vi "PlantModel.vi"(7 "error in (no error)":errorcluster, 8 "ROSCO Params in":T1, 9 "?":T2={"iSTATUS"=0, "TIME"=1, "DT"=2, "BL_PITCH_1"=3, "VS_MECHGENPWR"=13, "GEN_SPEED"=19, "ROT_SPEED"=20, "GENTQMEAS"=22, "Y_M"=23, "HORWINDV"=26, "ROOTMOOP1"=29, "ROOTMOOP2"=30, "BL_PITCH_2"=32, "BL_PITCH_3"=33, "ROOTMOOP3"=31, "INFILE_SIZE"=49, "FA_ACC"=52, "NUM_BLADES"=60, " OUT BL_PITCH"=44, "OUT_ TORQUE"=46, "OUTFILE_SIZE "=49, "AVCMSG_SIZE"=49, "AERODYN TQ"=89, "VS_GENPWR"=13}) -> (0 "error out":errorcluster, 1 "ROSCO Params out":T1, 3 "wdot/w":sgl)   [LabVIEW 2018]
uses:
  Clusters/RoscoParams.ctl
  Clusters/SwapIndexes.ctl
  Clusters/SimulationConstants.ctl
panel:
  out "element 4":sgl
  out "element 3":sgl
  out "element 2":sgl
  out "element":sgl
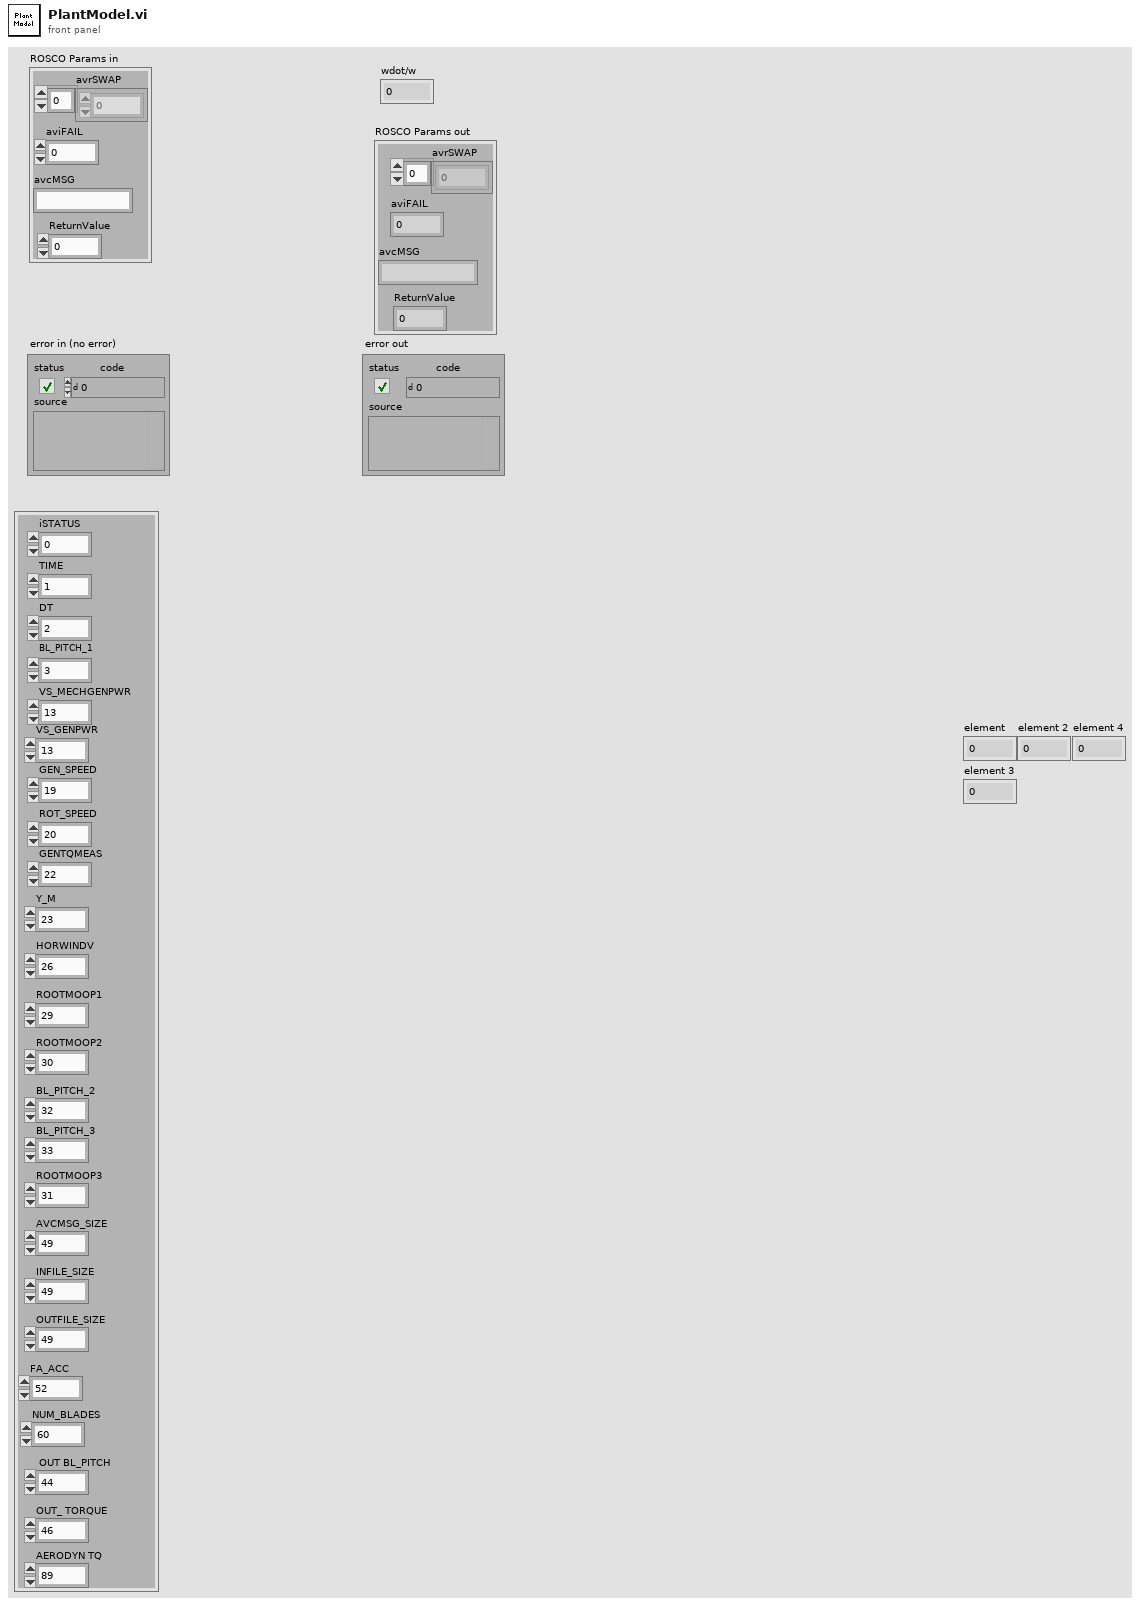
[diagram p1: front panel]
types:
  T1 = typedef "RoscoParams.ctl" = cluster{"avrSWAP":sgl[], "aviFAIL":i32, "avcMSG":string, "ReturnValue":i32}
  T2 = typedef "SwapIndexes.ctl" = cluster{"iSTATUS":i32, "TIME":i32, "DT":i32, "BL_PITCH_1":i32, "VS_MECHGENPWR":i32, "GEN_SPEED":i32, "ROT_SPEED":i32, "GENTQMEAS":i32, "Y_M":i32, "HORWINDV":i32, "ROOTMOOP1":i32, "ROOTMOOP2":i32, "BL_PITCH_2":i32, "BL_PITCH_3":i32, "ROOTMOOP3":i32, "INFILE_SIZE":i32, "FA_ACC":i32, "NUM_BLADES":i32, " OUT BL_PITCH":i32, "OUT_ TORQUE":i32, "OUTFILE_SIZE ":i32, "AVCMSG_SIZE":i32, "AERODYN TQ":i32, "VS_GENPWR":i32}
  T3 = typedef "SimulationConstants.ctl" = cluster{"Ngear":sgl, "RotorInertia":sgl, "GeneratorEff":sgl, "RotorRadius":sgl, "Rho":sgl}
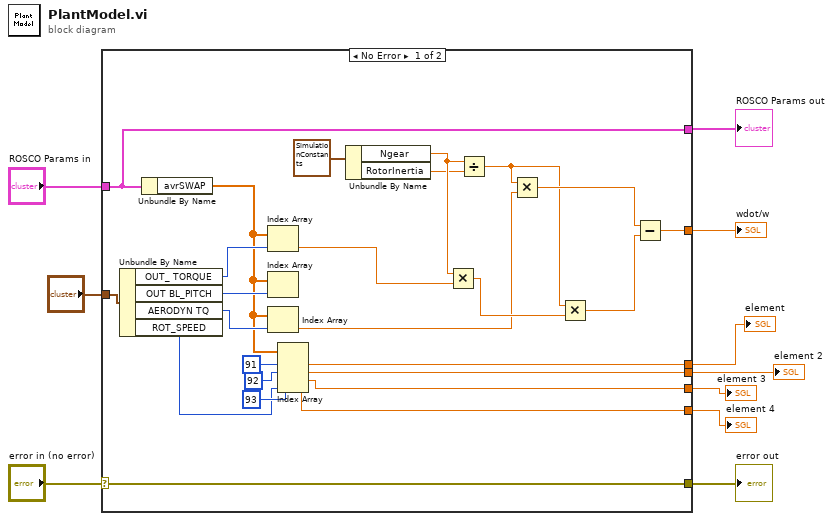
[diagram p0: block diagram]
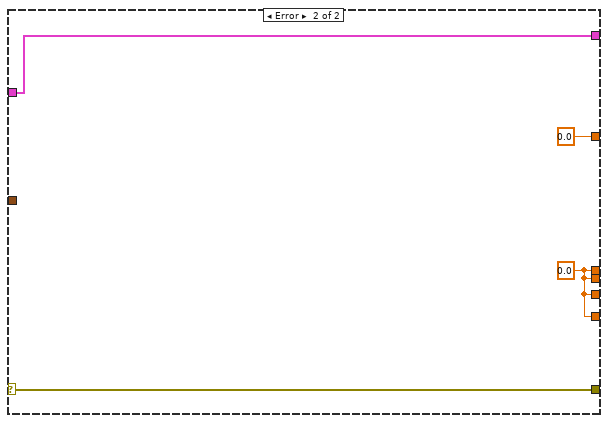
[diagram p2: hidden frame]
diagram:
  n1 = case shown="No Error" "error in (no error)" {
    selector: "error in (no error)" -> [w21 w38]
    tunnel: "ROSCO Params in" -> [w20 w37]
    tunnel: "?" -> [w23 _]
    tunnel: [w22 sgl 0.0] -> w8
    tunnel: [w21 w38] -> w6
    tunnel: [w20 w37] -> w5
    tunnel: [w17 w36] -> w4
    tunnel: [w16 w36] -> w3
    tunnel: [w13 w36] -> w2
    tunnel: [w11 w36] -> w1
    frame No Error {
      n2 = Unbundle By Name(w23) -> ("OUT_ TORQUE"=w24:i32, "OUT BL_PITCH"=w25:i32, "AERODYN TQ"=w26:i32, "ROT_SPEED"=w12:i32)
      n3 = Unbundle By Name(w20) -> ("avrSWAP"=w19:sgl[])
      n4 = Index Array(array=w19, index=w24) -> (element=w32:sgl)
      n5 = Index Array(array=w19, index=w25) -> ()  [unwired: 1 out]
      n6 = Index Array(array=w19, index=w26) -> (element=w29:sgl)
      n7 = Index Array(array=w19, index #1=91 ("index"), index #2=92 ("index"), index #3=93 ("index"), index #4=w12) -> (element #1=w17:sgl, element #2=w16:sgl, element #3=w13:sgl, element #4=w11:sgl)
      n8 = Unbundle By Name(T3 {"Ngear"=1.0, "RotorInertia"=318628130.0, "GeneratorEff"=318628130.0, "RotorRadius"=0.97, "Rho"=0.97}) -> ("Ngear"=w31:sgl, "RotorInertia"=w28:sgl)
      n9 = Multiply(x=w31, y=w32) -> (x*y=w33:sgl)
      n10 = Divide(x=w31, y=w28) -> (x/y=w30:sgl)
      n11 = Multiply(x=w30, y=w29) -> (x*y=w35:sgl)
      n12 = Multiply(x=w30, y=w33) -> (x*y=w34:sgl)
      n13 = Subtract(x=w35, y=w34) -> (x-y=w22:sgl)
    }
    frame Error {
      w36 = sgl 0.0 ("element")
    }
  }
  "wdot/w" <- w8
  "error out" <- w6
  "ROSCO Params out" <- w5
  "element" <- w4
  "element 2" <- w3
  "element 3" <- w2
  "element 4" <- w1
